vi "Sine Generator.vi"(1 "Blink Period (s)":dbl, 2 "Loop Rate (ms)":i64) -> (0 "Intensity (%)":dbl[](array[numeric]))   [LabVIEW 2016]
uses:
  <vilib>/Analysis/NI_AALBase.lvlib
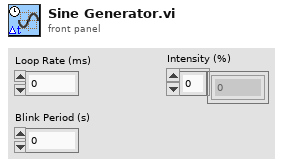
[diagram p1: front panel]
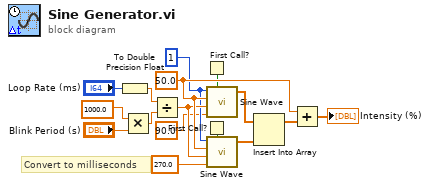
[diagram p0: block diagram]
diagram:
  w16 = 50.0 ("amplitude")
  w9 = 1 ("samples")
  # "Convert to milliseconds"
  n1 = To Double Precision Float(number="Loop Rate (ms)") -> (double precision float=w7:dbl)
  n2 = Multiply(x=1000.0, y="Blink Period (s)") -> (x*y=w3:dbl)
  n3 = Divide(x=w7, y=w3) -> (x/y=w10:dbl)
  n4 = First Call?() -> (First Call?: T/F=w2:bool)
  n5 = First Call?() -> (First Call?: T/F=w1:bool)
  n6 = call <vilib>:"Sine Wave.vi"("samples"=w9, "amplitude"=w16, "frequency"=w10, "phase in"=90.0, "reset phase"=w2) -> ("sine wave"=w12:dbl[])  [unwired: 2 out]
  n7 = call <vilib>:"Sine Wave.vi"("samples"=w9, "amplitude"=w16, "frequency"=w10, "phase in"=270.0, "reset phase"=w1) -> ("sine wave"=w13:dbl[])  [unwired: 2 out]
  n8 = Insert Into Array(array=w12, new element=w13) -> (w14:dbl[])  [unwired: 1 in]
  n9 = Add(x=w16, y=w14) -> (x+y=→"Intensity (%)":dbl[])
